vi "SMU Switch Handshaking - LV code improvements.vi"(8 "error in":errorcluster, 10 "Error Stream gRPCid":T1, 11 "file path (use dialog)":path=path "/home/lvuser/jsontestfile.json") -> (0 "error out":errorcluster, 1 "Results":T2[](array[typedef]), 3 "Elapsed Time":u32)   [LabVIEW 2019]
uses:
  labview-grpc-query-server/VIs/MeasurementServer_FourProbeRawData.ctl
  labview-grpc-query-server/VIs/MeasurementServer_ErrorOutData.ctl
  labview-grpc-query-server/VIs/MeasurementServer_gRPCid.ctl
  <instrlib>/niDCPower/nidcpower.llb/niDCPower Send Software Edge Trigger - Signal.ctl
  Global Operations.ctl
  <instrlib>/niDCPower/nidcpower.llb/niDCPower Wait For Event - Event.ctl
  <instrlib>/niDCPower/nidcpower.llb/niDCPower Configure Software Edge Start Trigger.vi
  <instrlib>/niDCPower/nidcpower.llb/niDCPower Configure Software Edge Sequence Advance Trigger.vi
  labview-grpc-query-server/VIs/labview-grpc-measurement-server.lvlib
  SupportVIs.lvlib
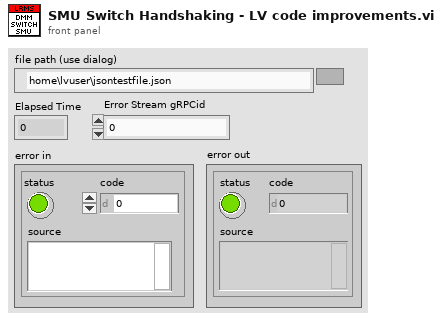
[diagram p1: front panel]
types:
  T1 = typedef "labview-grpc-measurement-server.lvlib/MeasurementServer_gRPCid.ctl" = u64
  T2 = typedef "labview-grpc-measurement-server.lvlib/MeasurementServer_FourProbeRawData.ctl" = cluster{"Positive Voltage":dbl, "Positive Current":dbl, "Negative Voltage":dbl, "Negative Current":dbl, "Impedance":dbl, "ErrorOutData":T3}
  T3 = typedef "labview-grpc-measurement-server.lvlib/MeasurementServer_ErrorOutData.ctl" = cluster{"ErrorCode":i32, "ErrorMessage":string}
  T4 = typedef "niDCPower Send Software Edge Trigger - Signal.ctl" = i32
  T5 = typedef "JSONCluster.ctl" = cluster{"SMUResourceName":string, "SMUChannels":string, "SMUSourceMode":i32, "SMUOutputFunction":i32, "SMUSourceTransientResponse":i32, "SMUCurrent":dbl, "SMUCurrentLevelRange":dbl, "SMUMeasurementSense":i32, "SMUMeasurementApertureTime":dbl, "SMUSourceAdvancedSourceDelay":dbl, "SMUVoltage":dbl, "SMUSourceAdvancedSequenceLoopCount":i32, "SMUMeasurementAdvancedDCNoiseRejection":i32, "SMUSequenceName":string, "SMUStep1_Source_DCCurrent_CurrentLevel":i32, "SMUStep2_Measurement_ApertureTime":i32, "SMUStep3_Source_Advanced_SourceDelay":i32, "SMUSequenceNumberOfSteps":i32, "ScanList":string, "Switch1ResourceName":string, "Switch1Topology":string, "Switch1ScanList":string, "Switch2ResourceName":string, "Switch2Topology":string, "Switch2ScanList":string, "DMMResourceName":string, "DMMFunction":i32, "DMMResolution":dbl, "DMMRange":dbl, "DMMSampleCount":i32, "DMMApertureTimeUnit":i32, "DMMApertureTime":dbl, "DMMNumberOfAverages":i32, "DMMAutoZero":i32, "DMMADCCalibration":i32, "DMMSettleTime":dbl, "DMMControlAction":i32, "DMMVoltageFaultUpperLimit":dbl, "ApplicationNumberOfWeldChannels":i32}
  T6 = typedef "Global Operations.ctl" = enum16{"Get", "Set"}
  T7 = typedef "niDMM Acquisition State.ctl" = enum16{"Running", "Finished with Backlog", "Finished with no Backlog", "Paused", "No acquisition in progress"}
  T8 = typedef "niDCPower Wait For Event - Event.ctl" = i32
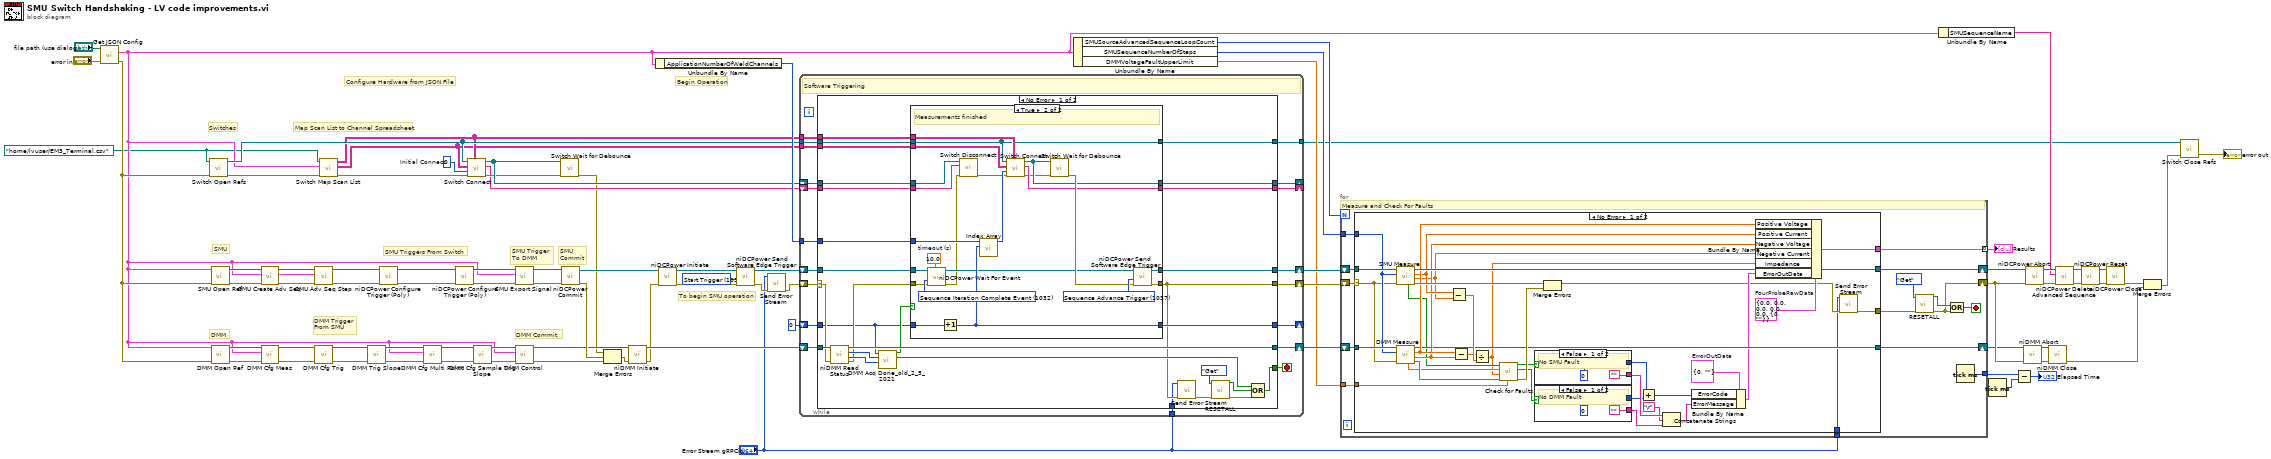
[diagram p0: block diagram]
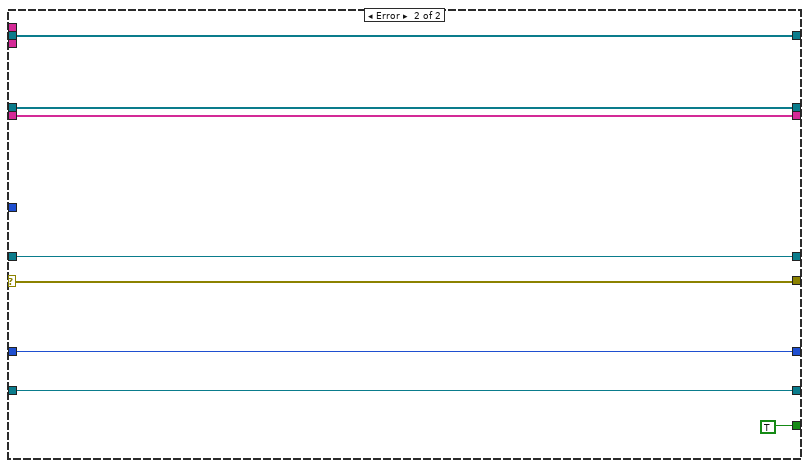
[diagram p3: hidden frame]
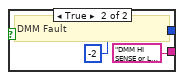
[diagram p4: hidden frame]
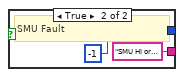
[diagram p5: hidden frame]
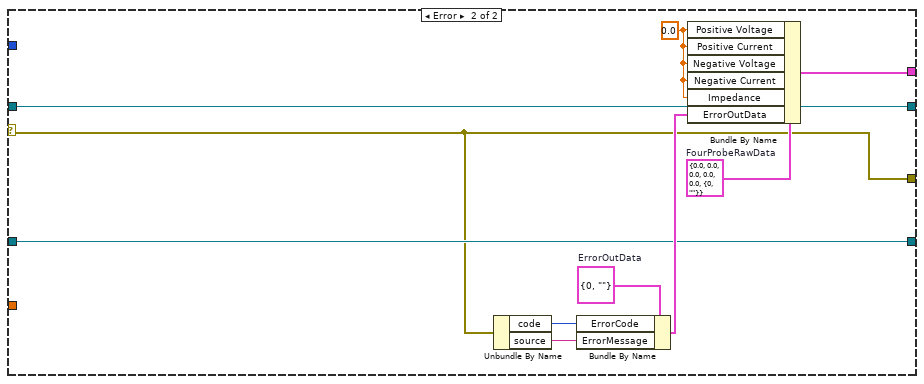
[diagram p6: hidden frame]
diagram:
  w1 = path "/home/lvuser/EM3_Terminal.csv" ("Ch Spreadsheet")
  w5 = 0  # Initial Connect
  w30 = T4 1034 items=["Start Trigger"=1034, "Source Trigger"=1035, "Measure Trigger"=1036, "Sequence Advance Trigger"=1037, "Pulse Trigger"=1053] ("signal")
  # "Map Scan List to Channel Spreadsheet"
  # "SMU\nCommit"
  # "DMM Commit"
  # "Begin Operation"
  # "Configure Hardware from JSON File"
  # "DMM"
  # "SMU"
  # "Switches"
  # "To begin SMU operation"
  # "DMM Trigger\nFrom SMU"
  # "SMU Trigger \nTo DMM"
  # "SMU Triggers From Switch"
  n1 = call "Get JSON Config.vi"("error in (no error)"="error in", "JSON Configuration File (.json)"="file path (use dialog)") -> ("error out"=w18:errorcluster, "JSONCluster"=w2:T5)  [unwired: 6 in, 2 out]
  n2 = call "Switch Open Refs.vi"("error in"=w18, "CSV File"=w1) -> ("error out"=w8:errorcluster, "Switch Refs"=w12:refnum<k15>[])  [unwired: 8 in]
  n3 = call "SMU Open Ref.vi"("error in (no error)"=w18, "JSONCluster"=w2) -> ("error out"=w81:errorcluster, "IVI Refnum out"=w82:refnum<k15>)  [unwired: 8 in]
  n4 = call "DMM Open Ref.vi"("error in"=w18, "JSONCluster"=w2) -> ("error out"=w54:errorcluster, "IVI Refnum out"=w53:refnum<k15>)  [unwired: 8 in]
  n5 = call "SMU Create Adv Seq.vi"("error in (no error)"=w81, "JSONCluster"=w2, "IVI Refnum in"=w82) -> ("error out"=w69:errorcluster, "IVI Refnum out"=w70:refnum<k15>)  [unwired: 7 in]
  n6 = call "DMM Cfg Meas.vi"("error in (no error)"=w54, "JSONCluster"=w2, "IVI Refnum in"=w53) -> ("error out"=w58:errorcluster, "IVI Refnum out"=w57:refnum<k15>)  [unwired: 7 in]
  n7 = call "SMU Adv Seq Step.vi"("error in (no error)"=w69, "JSONCluster"=w2, "IVI Refnum in"=w70) -> ("error out"=w67:errorcluster, "IVI Refnum out"=w68:refnum<k15>)  [unwired: 7 in]
  n8 = call "DMM Cfg Trig.vi"("error in (no error)"=w58, "IVI Refnum in"=w57) -> ("error out"=w60:errorcluster, "IVI Refnum out"=w59:refnum<k15>)  [unwired: 8 in]
  n9 = call "Switch Map Scan List.vi"("error in (no error)"=w8, "JSONCluster"=w2, "Ch Spreadsheet"=w1) -> ("error out"=w7:errorcluster, "IVI Specifications"=w10:string[][], "Channel Specs"=w11:string[][])  [unwired: 6 in]
  n10 = call "DMM Trig Slope.vi"("error in (no error)"=w60, "IVI Refnum in"=w59) -> ("error out"=w62:errorcluster, "IVI Refnum out"=w61:refnum<k15>)  [unwired: 8 in]
  n11 = call-poly <instrlib>:"niDCPower Configure Trigger (Poly).vi"("error in (no error)"=w67, "instrument handle"=w68) -> ("error out"=w78:errorcluster, "instrument handle out"=w79:refnum<k15>)  [unwired: 8 in]
  n12 = call "DMM Cfg Multi Point.vi"("error in (no error)"=w62, "JSONCluster"=w2, "IVI Refnum in"=w61) -> ("error out"=w64:errorcluster, "IVI Refnum out"=w63:refnum<k15>)  [unwired: 7 in]
  n13 = call-poly <instrlib>:"niDCPower Configure Trigger (Poly).vi"("error in (no error)"=w78, "instrument handle"=w79) -> ("error out"=w40:errorcluster, "instrument handle out"=w41:refnum<k15>)  [unwired: 8 in]
  n14 = call "Switch Connect.vi"("Channel Specs"=w11, "error in (no error)"=w7, "Channel Index"=w5, "IVI Specifications"=w10, "Switch Refs"=w12) -> ("error out"=w6:errorcluster, "Channels Connected"=w4:string[], "Refs Connected"=w13:refnum<k15>[])  [unwired: 4 in]
  n15 = call "DMM Cfg Sample Trig Slope.vi"("error in (no error)"=w64, "IVI Refnum in"=w63) -> ("error out"=w46:errorcluster, "IVI Refnum out"=w47:refnum<k15>)  [unwired: 8 in]
  n16 = call "SMU Export Signal.vi"("error in (no error)"=w40, "JSONCluster"=w2, "IVI Refnum in"=w41) -> ("error out"=w65:errorcluster, "IVI Refnum out"=w66:refnum<k15>)  [unwired: 7 in]
  n17 = call "DMM Control.vi"("error in (no error)"=w46, "JSONCluster"=w2, "IVI Refnum in"=w47) -> ("error out"=w51:errorcluster, "IVI Refnum out"=w48:refnum<k15>)  [unwired: 7 in]
  n18 = call "Switch Wait for Debounce.vi"("error in (no error)"=w6, "Switch Refs"=w13) -> ("error out"=w3:errorcluster)  [unwired: 9 in]
  n19 = call <instrlib>:"niDCPower Commit.vi"("error in (no error)"=w65, "instrument handle"=w66) -> ("error out"=w52:errorcluster, "instrument handle out"=w49:refnum<k15>)  [unwired: 8 in]
  n20 = Merge Errors(w3, w52, w51) -> (w50:errorcluster)
  n21 = call <instrlib>:"niDMM Initiate.vi"("error in (no error)"=w50, "instrument handle"=w48) -> ("error out"=w23:errorcluster, "instrument handle out"=w29:refnum<k15>)  [unwired: 8 in]
  n22 = Unbundle By Name(w2) -> ("ApplicationNumberOfWeldChannels"=w25:i32)
  n23 = call <instrlib>:"niDCPower Initiate.vi"("error in (no error)"=w23, "instrument handle"=w49) -> ("error out"=w24:errorcluster, "instrument handle out"=w32:refnum<k15>)  [unwired: 8 in]
  n24 = call <instrlib>:"niDCPower Send Software Edge Trigger.vi"("error in (no error)"=w24, "signal"=w30, "instrument handle"=w32) -> ("error out"=w16:errorcluster, "instrument handle out"=w31:refnum<k15>)  [unwired: 7 in]
  n25 = call "Send Error Stream.vi"("error in (no error)"=w16, "Error Stream gRPCid"="Error Stream gRPCid") -> ("error out"=w15:errorcluster)  [unwired: 9 in]
  n26 = while {
    shift-right: [w101] -> w34
    shift-left: w31 -> [w98]
    shift-right: [w99] -> w33
    shift-left: w15 -> [w92]
    shift-right: [w96] -> w28
    shift-left: w29 -> [w97]
    shift-right: [w94] -> _
    shift-left: 0 ("Backlog") -> [w95]
    tunnel: w25 -> [w93]
    tunnel: "Error Stream gRPCid" -> [w91]
    shift-right: [w87] -> _
    shift-left: w13 -> [w89]
    shift-right: [w86] -> _
    shift-left: w4 -> [w90]
    tunnel: w12 -> [w88]
    tunnel: w11 -> [w85]
    tunnel: w10 -> [w84]
    tunnel: [w83] -> w9
    stop <- w100 stop-if-true
    # "Software Triggering"
    n27 = case shown="No Error" w92 {
      selector: w92 -> [w119 w165]
      tunnel: [w129 w166] -> w101
      tunnel: [w114 TRUE] -> w100
      tunnel: [w113 w165] -> w99
      tunnel: w98 -> [w128 w166]
      tunnel: w97 -> [w125 w163]
      tunnel: [w124 w163] -> w96
      tunnel: w95 -> [w102 w164]
      tunnel: [w123 w164] -> w94
      tunnel: w93 -> [w121 _]
      tunnel: w91 -> [w112 _]
      tunnel: w90 -> [w109 w160]
      tunnel: w89 -> [w110 w161]
      tunnel: w88 -> [w108 w159]
      tunnel: [w107 w161] -> w87
      tunnel: [w106 w160] -> w86
      tunnel: w85 -> [w105 _]
      tunnel: w84 -> [w104 _]
      tunnel: [w103 w159] -> w83
      frame No Error {
        n28 = call <instrlib>:"niDMM Read Status.vi"("error in (no error)"=w119, "instrument handle"=w125) -> ("error out"=w120:errorcluster, "Acquisition State"=w127:T7, "Backlog"=w126:i32, "instrument handle out"=w124:refnum<k15>)  [unwired: 6 in]
        n29 = call "DMM Acq Done_old_2_5_2021.vi"("Acquisition State"=w127, "Backlog"=w126, "Channel Index"=w102) -> ("Finished with Backlog?"=w115:bool, "Sequence Acquision Finished?"=w122:bool)  [unwired: 7 in]
        n30 = case shown="True" w122 {
          tunnel: w120 -> [w134 w138]
          tunnel: [w135 w158] -> w129
          tunnel: [w134 w157] -> w113
          tunnel: w128 -> [w135 w140]
          tunnel: w102 -> [w133 w154]
          tunnel: [w133 w152] -> w123
          tunnel: w121 -> [_ w151]
          tunnel: w110 -> [w132 w149]
          tunnel: w109 -> [w131 w150]
          tunnel: w108 -> [w130 w144]
          tunnel: [w132 w148] -> w107
          tunnel: [w131 w147] -> w106
          tunnel: w105 -> [_ w146]
          tunnel: w104 -> [_ w145]
          tunnel: [w130 w144] -> w103
          frame False {
            # "Measurements not finished yet - repeat loop"
          }
          frame True {
            w136 = 10.0  # timeout (s)
            w141 = T8 1032 items=["Source Complete Event"=1030, "Measure Complete Event"=1031, "Sequence Iteration Complete Event"=1032, "Sequence Engine Done Event"=1033, "Pulse Complete Event"=1051, "Ready For Pulse Trigger Event"=1052] ("event")
            w156 = T4 1037 items=["Start Trigger"=1034, "Source Trigger"=1035, "Measure Trigger"=1036, "Sequence Advance Trigger"=1037, "Pulse Trigger"=1053] ("signal")
            # "Measurements finished"
            n31 = call <instrlib>:"niDCPower Wait For Event.vi"("timeout (sec)"=w136, "error in (no error)"=w138, "event"=w141, "instrument handle"=w140) -> ("error out"=w137:errorcluster, "instrument handle out"=w139:refnum<k15>)  [unwired: 6 in]
            n32 = Increment(x=w154) -> (x+1=w152:i32)
            n33 = call "Switch Disconnect.vi"("error in (no error)"=w137, "Channels Connected"=w150, "Switch Refs"=w149) -> ("error out"=w143:errorcluster)  [unwired: 8 in]
            n34 = call "Index Array.vi"("Backlog"=w152, "ApplicationNumberOfWeldChannels"=w151) -> ("Index"=w153:i32)  [unwired: 9 in]
            n35 = call "Switch Connect.vi"("Channel Specs"=w146, "error in (no error)"=w143, "Channel Index"=w153, "IVI Specifications"=w145, "Switch Refs"=w144) -> ("error out"=w142:errorcluster, "Channels Connected"=w147:string[], "Refs Connected"=w148:refnum<k15>[])  [unwired: 4 in]
            n36 = call "Switch Wait for Debounce.vi"("error in (no error)"=w142, "Switch Refs"=w148) -> ("error out"=w155:errorcluster)  [unwired: 9 in]
            n37 = call <instrlib>:"niDCPower Send Software Edge Trigger.vi"("error in (no error)"=w155, "signal"=w156, "instrument handle"=w139) -> ("error out"=w157:errorcluster, "instrument handle out"=w158:refnum<k15>)  [unwired: 7 in]
          }
        }
        n38 = call "Send Error Stream.vi"("error in (no error)"=w113, "Error Stream gRPCid"=w112) -> ("error out"=w111:errorcluster)  [unwired: 9 in]
        n39 = call "RESETALL.vi"("error in (no error)"=w111, "Operation"=Global_Operations."Get") -> ("error out"=w117:errorcluster, "RESETALL?"=w116:bool)  [unwired: 8 in]
        n40 = Compound Arithmetic op=OR(w115, w116, w117) -> (w114:bool)
      }
      frame Error {
      }
    }
  }
  n41 = Unbundle By Name(w2) -> ("SMUSourceAdvancedSequenceLoopCount"=w36:i32, "SMUSequenceNumberOfSteps"=w35:i32, "DMMVoltageFaultUpperLimit"=w17:dbl)
  n42 = for {
    N: w36 -> [_]
    tunnel: w35 -> [w178]
    shift-right: [w169] -> w45
    shift-left: w33 -> [w173]
    shift-right: [w181] -> w80
    shift-left: w34 -> [w179]
    shift-right: [w177] -> w42
    shift-left: w28 -> [w180]
    tunnel: [w176] -> w21 mode=indexing
    tunnel: [w175] -> w19
    tunnel: w17 -> [w174]
    tunnel: "Error Stream gRPCid" -> [w167]
    stop <- w170 stop-if-true
    # "Measure and Check For Faults"
    n43 = case shown="No Error" w173 {
      selector: w173 -> [w185 w225]
      tunnel: [w216 w227] -> w181
      tunnel: w180 -> [w215 w226]
      tunnel: w179 -> [w209 w227]
      tunnel: w178 -> [w208 _]
      tunnel: [w203 w226] -> w177
      tunnel: [w201 w229] -> w176
      tunnel: w174 -> [w186 _]
      tunnel: [w183 w225] -> w168
      tunnel: w167 -> [w182 _]
      frame No Error {
        w188 = T3 {"ErrorCode"=0, "ErrorMessage"=""}  # ErrorOutData
        w187 = T2 {"Positive Voltage"=0.0, "Positive Current"=0.0, "Negative Voltage"=0.0, "Negative Current"=0.0, "Impedance"=0.0, "ErrorOutData"={"ErrorCode"=0, "ErrorMessage"=""}}  # FourProbeRawData
        n44 = call "SMU Measure.vi"("error in (no error)"=w185, "SMUSequenceNumberOfSteps"=w208, "IVI Refnum in"=w209) -> ("error out"=w214:errorcluster, "Numeric"=w204:dbl, "Numeric 2"=w206:dbl, "IVI Refnum out"=w216:refnum<k15>, "in compliance"=w191:bool[])  [unwired: 4 in]
        n45 = call "DMM Measure.vi"("error in (no error)"=w185, "SMUSequenceNumberOfSteps"=w208, "IVI Refnum in"=w215) -> ("error out"=w213:errorcluster, "Numeric"=w205:dbl, "Numeric 2"=w207:dbl, "IVI Refnum out"=w203:refnum<k15>, "Measurements"=w190:dbl[])  [unwired: 4 in]
        n46 = Subtract(x=w206, y=w204) -> (x-y=w211:dbl)
        n47 = Subtract(x=w207, y=w205) -> (x-y=w210:dbl)
        n48 = Divide(x=w210, y=w211) -> (x/y=w189:dbl)
        n49 = call "Check for Faults.vi"("DMM Voltage Fault Upper Limit"=w186, "Error In"=w213, "Resistance In"=w189, "dmm voltage measurements"=w190, "in compliance"=w191) -> ("Error Out"=w212:errorcluster, "DMM Fault"=w195:bool, "SMU Fault"=w199:bool)  [unwired: 3 in, 1 out]
        n50 = case shown="False" w199 {
          tunnel: ["" "SMU HI or LO lead disconnected\n- SMU in compliance\n- SMU Fault = True"] -> w198
          tunnel: [0 -1] -> w196
          frame False {
            # "No SMU Fault"
          }
          frame True {
            # "SMU Fault"
          }
        }
        n51 = case shown="False" w195 {
          tunnel: ["" "DMM HI SENSE or LO SENSE lead disconnected\n- DMM measures NaN, or \n- DMM overrange warning, or\n- DMM voltage > 50uV "] -> w193
          tunnel: [0 -2] -> w192
          frame False {
            # "No DMM Fault"
          }
          frame True {
            # "DMM Fault"
          }
        }
        n52 = Merge Errors(w214, w212) -> (w184:errorcluster)
        n53 = Add(x=w196, y=w192) -> (x+y=w200:i32)
        n54 = Concatenate Strings(w198, "\r", w193) -> (w197:string)
        n55 = Bundle By Name(cluster=w188, "ErrorCode"=w200, "ErrorMessage"=w197) -> (w202:T3)
        n56 = Bundle By Name(cluster=w187, "Positive Voltage"=w207, "Positive Current"=w206, "Negative Voltage"=w205, "Negative Current"=w204, "Impedance"=w189, "ErrorOutData"=w202) -> (w201:T2)
        n57 = call "Send Error Stream.vi"("error in (no error)"=w184, "Error Stream gRPCid"=w182) -> ("error out"=w183:errorcluster)  [unwired: 9 in]
      }
      frame Error {
        w228 = 0.0 ("Positive Voltage")
        w232 = T3 {"ErrorCode"=0, "ErrorMessage"=""}  # ErrorOutData
        w233 = T2 {"Positive Voltage"=0.0, "Positive Current"=0.0, "Negative Voltage"=0.0, "Negative Current"=0.0, "Impedance"=0.0, "ErrorOutData"={"ErrorCode"=0, "ErrorMessage"=""}}  # FourProbeRawData
        n58 = Unbundle By Name(w225) -> ("code"=w230:i32, "source"=w231:string)
        n59 = Bundle By Name(cluster=w232, "ErrorCode"=w230, "ErrorMessage"=w231) -> (w234:T3)
        n60 = Bundle By Name(cluster=w233, "Positive Voltage"=w228, "Positive Current"=w228, "Negative Voltage"=w228, "Negative Current"=w228, "Impedance"=w228, "ErrorOutData"=w234) -> (w229:T2)
      }
    }
    n61 = call "RESETALL.vi"("error in (no error)"=w168, "Operation"=Global_Operations."Get") -> ("error out"=w169:errorcluster, "RESETALL?"=w171:bool)  [unwired: 8 in]
    n62 = Compound Arithmetic op=OR(w171, w169) -> (w170:bool)
    n63 = Tick Count (ms)() -> (millisecond timer value=w175:u32)
  }
  "Results" <- w21
  n64 = Unbundle By Name(w2) -> ("SMUSequenceName"=w20:string)
  n65 = Tick Count (ms)() -> (millisecond timer value=w77:u32)
  n66 = Subtract(x=w19, y=w77) -> (x-y=→"Elapsed Time":u32)
  n67 = call <instrlib>:"niDMM Abort.vi"("error in (no error)"=w45, "instrument handle"=w42) -> ("error out"=w56:errorcluster, "instrument handle out"=w55:refnum<k15>)  [unwired: 8 in]
  n68 = call <instrlib>:"niDCPower Abort.vi"("error in (no error)"=w45, "instrument handle"=w80) -> ("error out"=w75:errorcluster, "instrument handle out"=w76:refnum<k15>)  [unwired: 8 in]
  n69 = call <instrlib>:"niDMM Close.vi"("error in (no error)"=w56, "instrument handle"=w55) -> ("error out"=w44:errorcluster)  [unwired: 9 in]
  n70 = call <instrlib>:"niDCPower Delete Advanced Sequence.vi"("error in (no error)"=w75, "sequence name"=w20, "instrument handle"=w76) -> ("error out"=w74:errorcluster, "instrument handle out"=w73:refnum<k15>)  [unwired: 7 in]
  n71 = call <instrlib>:"niDCPower Reset.vi"("error in (no error)"=w74, "instrument handle"=w73) -> ("error out"=w71:errorcluster, "instrument handle out"=w72:refnum<k15>)  [unwired: 2 in, 6 out]
  n72 = call <instrlib>:"niDCPower Close.vi"("error in (no error)"=w71, "instrument handle"=w72) -> ("error out"=w43:errorcluster)  [unwired: 9 in]
  n73 = Merge Errors(w43, w44) -> (w26:errorcluster)
  n74 = call "Switch Close Refs.vi"("error in (no error)"=w26, "Switch Refs"=w9) -> ("error out"=→"error out":errorcluster)  [unwired: 9 in]
